vi "Database Path.vi"(8 "error in (no error)":errorcluster, 10 "Database Name (\"main\")":string="main", 11 "Connection in":refnum<class "Connection.lvclass">) -> (0 "error out":errorcluster, 2 "Path to Database":path, 3 "Connection out":refnum<class "Connection.lvclass">)   [LabVIEW 2011, in "SQLite.lvlib" / "Connection.lvclass"]
doc: "Returns the path to the database corresponding to the provided name. The main database of the connection has the name \"main\". Attached databases have names defined when added via the \"ATTACH\" SQL command. Temporary or in-memory databases return an empty path."
uses:
  Connection.lvclass
  Connection.lvclass/Connection.ctl
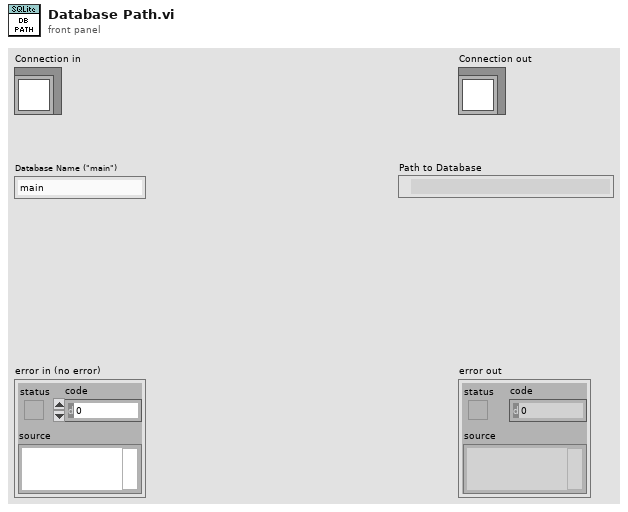
[diagram p1: front panel]
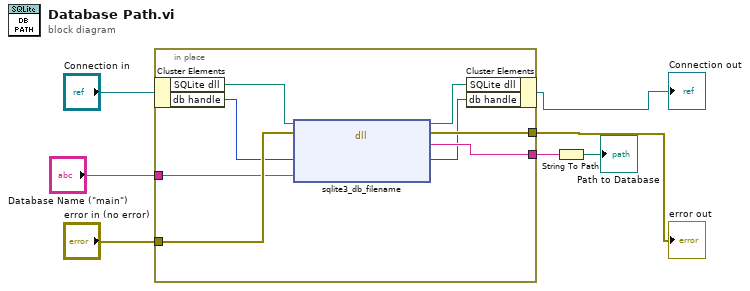
[diagram p0: block diagram]
diagram:
  n1 = in-place {
    in-place-border: "error in (no error)" -> [w15]
    in-place-border: "Database Name (\"main\")" -> [w14]
    in-place-border: [w13] -> w5
    in-place-border: [w12] -> w2
    n2 = in-place-cluster #1("Connection in") -> ("SQLite dll"=w8:path, "db handle"=w11:u64)
    n3 = dll-call lib="C:/drjdpowell/sqlite-labview/SQL Connection/sqlite3.dll" fn="sqlite3_db_filename"(path in=w8, error in=w15, "db"=w11, "name"=w14) -> (path out=w9:path, error out=w13:errorcluster, "filename"=w12:string, "db"=w10:u64)  [unwired: 2 in]
    n4 = in-place-cluster #1("SQLite dll"=w9, "db handle"=w10) -> (→"Connection out":refnum<class "Connection.lvclass">)
  }
  "error out" <- w5
  n5 = String To Path(string=w2) -> (path=→"Path to Database":path)
